vi "Init Actor Core.vi"(8 "error in (no error)":errorcluster, 11 "Measure Object in":refnum<class "Template Module.lvclass">) -> (0 "error out":errorcluster, 3 "Measure Object out":refnum<class "Template Module.lvclass">)   [LabVIEW 2016, in "Template Module.lvclass"]
uses:
  Template Module.lvclass
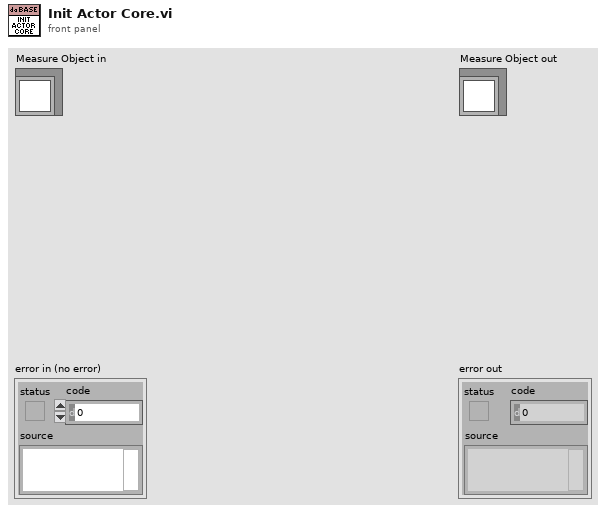
[diagram p1: front panel]
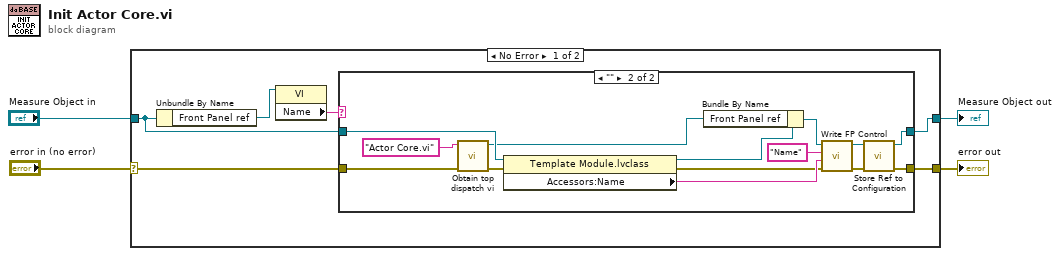
[diagram p0: block diagram]
diagram:
  n1 = case shown="No Error" "error in (no error)" {
    selector: "error in (no error)" -> [w8 w28]
    tunnel: [w7 w28] -> w3
    tunnel: [w5 w27] -> w1
    tunnel: "Measure Object in" -> [w6 w27]
    frame No Error {
      n2 = Unbundle By Name(w6) -> ("Front Panel ref"=w10:refnum<vi>)
      n3 = property class="VI"(reference=w10) -> ("Name"=w9:string)  [unwired: 1 in, 2 out]
      n4 = case shown="\"\"" w9 {
        tunnel: w8 -> [w12 w25]
        tunnel: w6 -> [w11 w24]
        tunnel: [w12 w14] -> w7
        tunnel: [w11 w15] -> w5
        frame Default {
        }
        frame "" {
          n5 = call "Obtain top dispatch vi.vi"("Error In"=w25, "VI name"="Actor Core.vi") -> ("Error Out"=w17:errorcluster, "vi reference"=w23:refnum<vi>)  [unwired: 7 in, 1 out]
          n6 = property class="Template Module.lvclass"(reference=w24, error in=w17) -> (reference out=w19:refnum<class "Template Module.lvclass">, error out=w16:errorcluster, "Accessors:Name"=w18:string)
          n7 = Bundle By Name(cluster=w19, "Front Panel ref"=w23) -> (w22:refnum<class "Template Module.lvclass">)
          n8 = call-dynamic "Write FP Control.vi"("error in (no error)"=w16, "Control Value"=w18, "Control Name"="Name", "Measure Object in"=w22) -> ("error out"=w13:errorcluster, "Measure Object out"=w21:refnum<class "Template Module.lvclass">)  [unwired: 6 in]
          n9 = call-dynamic "Store Ref to Configuration.vi"("error in (no error)"=w13, "Measure Object in"=w21) -> ("error out"=w14:errorcluster, "Measure Object out"=w15:refnum<class "Template Module.lvclass">)  [unwired: 8 in]
        }
      }
    }
    frame Error {
    }
  }
  "error out" <- w3
  "Measure Object out" <- w1
